vi "Bundle AOL parameters.vi"(10 "AOL_Globals in":T1={"Imaging Protocol"=enum."AOL Z-Stack", "Number of POI"=0, "Number of Miniscans"=0, "Number of Trials"=0, "Number of Cycles "=0, "# Averaged Frames"=0, "Laser power (%)"=0, "Pockels"=0.0, "Acquisition Length (sec)"=0.0, "Fill time (us)"=0.0, "POI Dwell time (us)"=0.0, "Miniscan Dwell time per pixel (us)"=0.0, "PMT 1"=0.0, "PMT 2"=0.0, "Back Apperture"=0.0, "Frame Size"=0, "Center Frequency"=0.0, "Field of View"=0.0, "DwellTime (us)"=0.0, "Wavelength (nm)"=0.0, "Zoom"=0.0, "AOL Z"=0.0, "AOL Mode"=enum."Raster", "GridXY"=0.0, "GridZ"=0.0, "TriggerPeriod (sec)"=0.0, "Number of Pixels in Miniscan"=0, "Experiment folder path"=path "", "X centre"=0.0, "Y centre"=0.0, "Angle (degrees)"=0.0, "Plane Mode"=0, "Threshold"=[], "Regenerate Chirps"=FALSE, "Rectangle ROI length (pixels)"=0, "Rectangle ROI height (pixels)"=0, "AOD fill"=0, "Samples Wait after Trigger"=0, "StartUp Delay"=0, "Slip Cycle"=163840, "Add Cycle"=FALSE} {"Plane Mode" items=["XY Plane"]; "Frame Size" items=["100X100"=100, "128X128"=128, "200X200"=200, "256X256"=256, "512X512"=512, "1024x1024"=1024, "2048x2048"=2048]; "Back Apperture" format="%#.6g"; "Pockels" format="%#.6g"; "PMT 2" format="%#.6g"; "PMT 1" format="%#.6g"; "Angle (degrees)" format="%#.6g"; "POI Dwell time (us)" format="%#.6g"}, 11 "Experiment folder path":path) -> (3 "AOL_Globals out":T1={"Imaging Protocol"=enum."AOL Z-Stack", "Number of POI"=0, "Number of Miniscans"=0, "Number of Trials"=0, "Number of Cycles "=0, "# Averaged Frames"=0, "Laser power (%)"=0, "Pockels"=0.0, "Acquisition Length (sec)"=0.0, "Fill time (us)"=0.0, "POI Dwell time (us)"=0.0, "Miniscan Dwell time per pixel (us)"=0.0, "PMT 1"=0.0, "PMT 2"=0.0, "Back Apperture"=0.0, "Frame Size"=0, "Center Frequency"=0.0, "Field of View"=0.0, "DwellTime (us)"=0.0, "Wavelength (nm)"=0.0, "Zoom"=0.0, "AOL Z"=0.0, "AOL Mode"=enum."Raster", "GridXY"=0.0, "GridZ"=0.0, "TriggerPeriod (sec)"=0.0, "Number of Pixels in Miniscan"=0, "Experiment folder path"=path "", "X centre"=0.0, "Y centre"=0.0, "Angle (degrees)"=0.0, "Plane Mode"=0, "Threshold"=[], "Regenerate Chirps"=FALSE, "Rectangle ROI length (pixels)"=0, "Rectangle ROI height (pixels)"=0, "AOD fill"=0, "Samples Wait after Trigger"=0, "StartUp Delay"=0, "Slip Cycle"=163840, "Add Cycle"=FALSE} {"Plane Mode" items=["XY Plane"]; "Frame Size" items=["100X100"=100, "128X128"=128, "200X200"=200, "256X256"=256, "512X512"=512, "1024x1024"=1024, "2048x2048"=2048]; "Back Apperture" format="%#.6g"; "Pockels" format="%#.6g"; "PMT 2" format="%#.6g"; "PMT 1" format="%#.6g"; "Angle (degrees)" format="%#.6g"; "POI Dwell time (us)" format="%#.6g"})   [LabVIEW 2013]
uses:
  Typedefs/Controls/AOL_Globals.ctl
  Typedefs/Imaging Protocols enum.ctl
  Typedefs/Frame Size.ctl
  Typedefs/AOL modes.ctl
  Typedefs/Plane Mode.ctl
  Global Variables/General Globals.vi
  Global Variables/gl_UI Ctrl Refs.vi
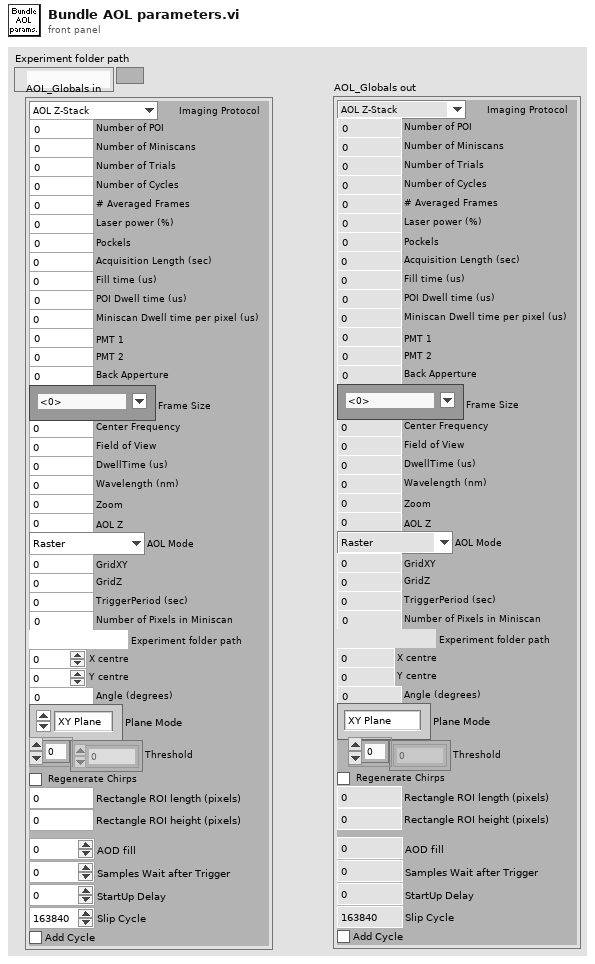
[diagram p1: front panel]
types:
  T1 = typedef "AOL_Globals.ctl" = cluster{"Imaging Protocol":T2, "Number of POI":u16, "Number of Miniscans":u16, "Number of Trials":u16, "Number of Cycles ":u64, "# Averaged Frames":u16, "Laser power (%)":u8, "Pockels":dbl, "Acquisition Length (sec)":dbl, "Fill time (us)":dbl, "POI Dwell time (us)":dbl, "Miniscan Dwell time per pixel (us)":dbl, "PMT 1":dbl, "PMT 2":dbl, "Back Apperture":dbl, "Frame Size":T3, "Center Frequency":dbl, "Field of View":dbl, "DwellTime (us)":dbl, "Wavelength (nm)":dbl, "Zoom":dbl, "AOL Z":dbl, "AOL Mode":T4, "GridXY":dbl, "GridZ":dbl, "TriggerPeriod (sec)":dbl, "Number of Pixels in Miniscan":u16, "Experiment folder path":path, "X centre":dbl, "Y centre":dbl, "Angle (degrees)":dbl, "Plane Mode":T5, "Threshold":u16[], "Regenerate Chirps":bool, "Rectangle ROI length (pixels)":u16, "Rectangle ROI height (pixels)":u16, "AOD fill":u16, "Samples Wait after Trigger":u16, "StartUp Delay":i32, "Slip Cycle":u32, "Add Cycle":bool}
  T2 = typedef "Imaging Protocols enum.ctl" = enum16{"AOL Z-Stack", "Motor Z Stack", "Functional Acquisition", "Single Plane Acquisition", "Volume Acquisition", "Live Imaging", "Live Plane Imaging", "Live Volume Imaging"}
  T3 = typedef "Frame Size.ctl" = u16
  T4 = typedef "AOL modes.ctl" = enum16{"Raster", "Structural", "Pointing", "Mini Scan", "Alignment"}
  T5 = typedef "Plane Mode.ctl" = u16
  T6 = typedef "UI ctrl refs cluster.ctl" = cluster{"Top level VI path":path, "Top level VI ref":refnum<vi>, "User menu ref":refnum<k9>, "Sub Panel control":refnum<vi>, "Imaging Param Tab":refnum<vi>, "Occurrence-Start drivers":refnum<k4>, "Occurrence-Speed logging initialised":refnum<k4>, "Occurrence-XYZ stage initialised":refnum<k4>, "Exit button":refnum<vi>, "Status ind":refnum<vi>, "Return to Origin":refnum<vi>, "Speed Logging":refnum<vi>, "Time Lapse":refnum<vi>, "Live Imaging":refnum<vi>, "AOL Z Stack":refnum<vi>, "Motor Z Stack":refnum<vi>, "Funct Acq button":refnum<vi>, "Hard Shutter":refnum<vi>, "Virtual Shutter":refnum<vi>, "Laser Power":refnum<vi>, "AOL Mode":refnum<vi>, "Frame Size":refnum<vi>, "Field of View":refnum<vi>, "Dwell Time":refnum<vi>, "Zoom":refnum<vi>, "AOL Z":refnum<vi>, "Objective":refnum<vi>, "Axis":refnum<vi>, "Paths & Names":refnum<vi>, "Experiment folder path (ind.)":refnum<vi>, "Last State (Ind.)":refnum<vi>, "Laser wavelength ind (nm)":refnum<vi>, "Averages":refnum<vi>, "Angle (degrees)":refnum<vi>, "X centre":refnum<vi>, "Y centre":refnum<vi>, "Plane Mode":refnum<vi>, "# Planes":refnum<vi>, "Z Start":refnum<vi>, "Z Stop":refnum<vi>, "Z Step":refnum<vi>, "PMT 1":refnum<vi>, "PMT 2":refnum<vi>, "Stage XYZ Position":refnum<vi>, "Pockels@Z Start":refnum<vi>, "Pockels@Z Stop":refnum<vi>, "Obtain Z Start":refnum<vi>, "Obtain Z Stop":refnum<vi>, "Live stim.trig.period":refnum<vi>, "Live stim.trig.enable":refnum<vi>, "Funct. Acq. Pockels Modulation":refnum<vi>, "Enable Video Recording":refnum<vi>, "Video Record-Live Imaging":refnum<vi>, "Video Record-Funct acq":refnum<vi>, "AOL Z-stack Chirps Ready (ind)":refnum<vi>, "Center freq ind (nm)":refnum<vi>, "Logging queue (ind)":refnum<vi>, "Back aperture power (ind.)":refnum<vi>, "Power after objective (ind.)":refnum<vi>, "Switch user":refnum<vi>}
  T7 = typedef "Laser control knob.ctl" = u16
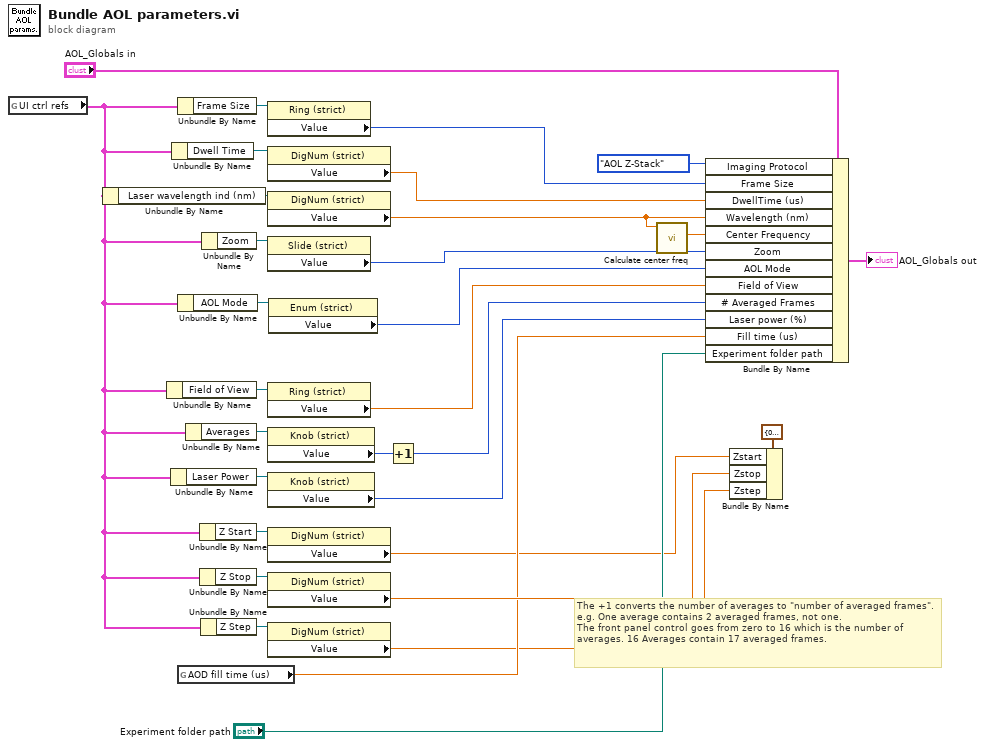
[diagram p0: block diagram]
diagram:
  # "The +1 converts the number of averages to \"number of averaged frames\". e.g. One average contains 2 averaged frames, not one.\nThe front panel control goes from zero to 16 which is the number of averages. 16 Averages contain 17 averaged frames."
  n1 = global read "gl_UI Ctrl Refs.vi" "UI ctrl refs"() -> (w5:T6)
  n2 = Unbundle By Name(w5) -> ("Laser wavelength ind (nm)"=w12:refnum<vi>)
  n3 = Unbundle By Name(w5) -> ("Field of View"=w13:refnum<vi>)
  n4 = Unbundle By Name(w5) -> ("Laser Power"=w27:refnum<vi>)
  n5 = Unbundle By Name(w5) -> ("Dwell Time"=w10:refnum<vi>)
  n6 = Unbundle By Name(w5) -> ("Frame Size"=w8:refnum<vi>)
  n7 = Unbundle By Name(w5) -> ("AOL Mode"=w4:refnum<vi>)
  n8 = global read "General Globals.vi" "AOD fill time (us)"() -> (w30:dbl)
  n9 = Unbundle By Name(w5) -> ("Averages"=w14:refnum<vi>)
  n10 = Unbundle By Name(w5) -> ("Z Start"=w20:refnum<vi>)
  n11 = Unbundle By Name(w5) -> ("Z Stop"=w19:refnum<vi>)
  n12 = Unbundle By Name(w5) -> ("Z Step"=w18:refnum<vi>)
  n13 = Unbundle By Name(w5) -> ("Zoom"=w11:refnum<vi>)
  n14 = property class="Ring (strict)"(reference=w8) -> ("Value"=w9:u16)  [unwired: 1 in, 2 out]
  n15 = property class="DigNum (strict)"(reference=w10) -> ("Value"=w15:dbl)  [unwired: 1 in, 2 out]
  n16 = property class="DigNum (strict)"(reference=w12) -> ("Value"=w1:dbl)  [unwired: 1 in, 2 out]
  n17 = property class="Slide (strict)"(reference=w11) -> ("Value"=w21:i8)  [unwired: 1 in, 2 out]
  n18 = property class="Ring (strict)"(reference=w13) -> ("Value"=w16:sgl)  [unwired: 1 in, 2 out]
  n19 = property class="Knob (strict)"(reference=w14) -> ("Value"=w17:u16)  [unwired: 1 in, 2 out]
  n20 = property class="Knob (strict)"(reference=w27) -> ("Value"=w28:T7)  [unwired: 1 in, 2 out]
  n21 = property class="DigNum (strict)"(reference=w20) -> ("Value"=w22:dbl)  [unwired: 1 in, 2 out]
  n22 = property class="DigNum (strict)"(reference=w19) -> ("Value"=w31:dbl)  [unwired: 1 in, 2 out]
  n23 = property class="DigNum (strict)"(reference=w18) -> ("Value"=w23:dbl)  [unwired: 1 in, 2 out]
  n24 = property class="Enum (strict)"(reference=w4) -> ("Value"=w3:T4)  [unwired: 1 in, 2 out]
  n25 = Increment(x=w17) -> (x+1=w29:u16)
  n26 = call "Calculate center freq.vi"("UI Wavelength"=w1) -> ("Centre frequency (MHz)"=w2:dbl)  [unwired: 9 in, 1 out]
  n27 = Bundle By Name(cluster="AOL_Globals in", "Imaging Protocol"=Imaging_Protocols_enum."AOL Z-Stack" ("Imaging Mode"), "Frame Size"=w9, "DwellTime (us)"=w15, "Wavelength (nm)"=w1, "Center Frequency"=w2, "Zoom"=w21, "AOL Mode"=w3, "Field of View"=w16, "# Averaged Frames"=w29, "Laser power (%)"=w28, "Fill time (us)"=w30, "Experiment folder path"="Experiment folder path") -> (→"AOL_Globals out":T1)
  n28 = Bundle By Name(cluster=cluster{"Zstart":dbl, "Zstop":dbl, "Zstep":dbl} {"Zstart"=0.0, "Zstop"=0.0, "Zstep"=0.0} ("ZStack"), "Zstart"=w22, "Zstop"=w31, "Zstep"=w23) -> ()  [unwired: 1 out]
